vi "ROI entry-Get dwell time from UI.vi"(1 "ROI Enum":T1) -> (0 "Dynamic dwell time(us)":dbl)   [LabVIEW 2020]
uses:
  Typedefs/ROI ID Enum.ctl
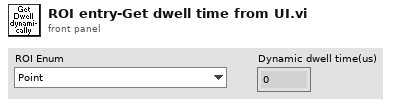
[diagram p1: front panel]
types:
  T1 = typedef "ROI ID Enum.ctl" = enum16{"Point", "MiniScan", "Comp. MiniScan", "Rectangle", "Comp. volume", "Arb. plane point", "None"}
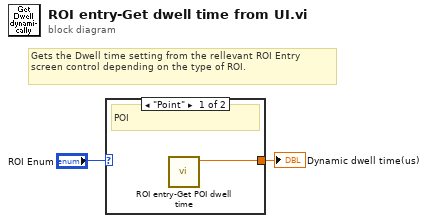
[diagram p0: block diagram]
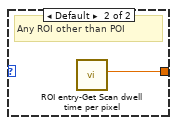
[diagram p2: hidden frame]
diagram:
  # "Gets the Dwell time setting from the rellevant ROI Entry screen control depending on the type of ROI."
  n1 = case shown="\"Point\"" "ROI Enum" {
    tunnel: [w3 w4] -> w2
    frame "Point" {
      # "POI"
      n2 = call "ROI entry-Get POI dwell time.vi"() -> ("POI Dwell time (us)"=w3:dbl)  [unwired: 10 in, 1 out]
    }
    frame Default {
      # "Any ROI other than POI"
      n3 = call "ROI entry-Get Scan dwell time per pixel.vi"() -> ("Scan dwell time per pixel (us)"=w4:dbl)  [unwired: 10 in, 1 out]
    }
  }
  "Dynamic dwell time(us)" <- w2
